vi "Close References.vi"(8 "error in (no error)":errorcluster, 11 "Setter Generator In":refnum<class "Setter Generator.lvclass">) -> (0 "error out":errorcluster)   [LabVIEW 2020, in "Method Generation.lvlib" / "Setter Generator.lvclass"]
uses:
  Setter Generator.lvclass
  Setter Generator.lvclass/Setter Generator.ctl
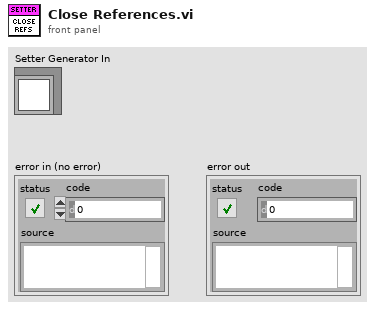
[diagram p1: front panel]
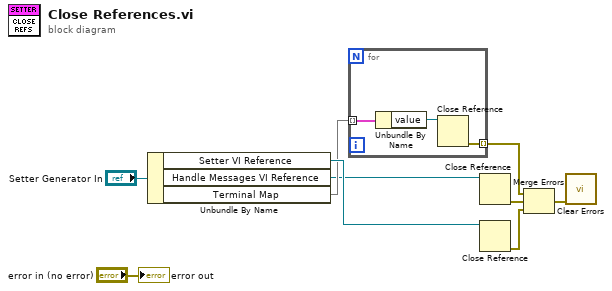
[diagram p0: block diagram]
diagram:
  n1 = Unbundle By Name("Setter Generator In") -> ("Setter VI Reference"=w8:refnum<vi>, "Handle Messages VI Reference"=w4:refnum<vi>, "Terminal Map"=w6:map{string, refnum<vi>})
  n2 = for {
    tunnel: w6 -> [w12] mode=indexing
    tunnel: [w10] -> w2 mode=indexing
    n3 = Unbundle By Name(w12) -> ("value"=w11:refnum<vi>)
    n4 = Close Reference(reference=w11) -> (error out=w10:errorcluster)  [unwired: 1 in]
  }
  n5 = Close Reference(reference=w4) -> (error out=w3:errorcluster)  [unwired: 1 in]
  n6 = Close Reference(reference=w8) -> (error out=w7:errorcluster)  [unwired: 1 in]
  n7 = Merge Errors(w2, w3, w7) -> (w1:errorcluster)
  n8 = call <vilib>:"Clear Errors.vi"("error in (no error)"=w1) -> ()  [unwired: 5 in, 2 out]
  "error out" <- "error in (no error)"
